vi "Single Tone Measurements.vi"(0 "scaled signals [EU]":waveform(dbl), 1 "tone detected":bool, 5 "frequency range":T1, 7 "window":T2 items=["None"=0, "Hanning"=1, "Hamming"=2, "Blackman-Harris"=3, "Exact Blackman"=4, "Blackman"=5, "Flat Top"=6, "4 Term B-Harris "=7, "7 Term B-Harris"=8, "Low Sidelobe"=9, "Force"=64, "Exponential"=65, "Blackman Nuttall"=11, "Triangle"=30, "Bartlett-Hanning"=31, "Bohman"=32, "Parzen"=33, "Welch"=34, "Kaiser"=60, "Dolph-Chebyshev"=61, "Gaussian"=62], 9 "Maximum Harmonic":i32, 11 "error in":errorcluster, 12 "Expected Frequency (Hz)":dbl) -> (4 "single-tone measurements":waveform(dbl)[](array[waveform]), 15 "error out":errorcluster)   [LabVIEW 2025, in "Tone Measurements.lvlib" / "Tone Measurements.lvclass"]
uses:
  Tone Measurements.lvclass
  <vilib>/addons/_NISVFA/_Shared subVIs/Controls/svc_Window.ctl
  <vilib>/addons/Sound and Vibration/svt_Level/SVL AC & DC Level (Time) (1 Ch).vi
  <vilib>/addons/Sound and Vibration/svt_Single Tone Measurements/SVT Spurious Free Dynamic Range (Frequency) (1 Ch).vi
  <vilib>/addons/_NISVFA/_Spectrum Processing/SVFA Unit Conversion (Complex) (1 Ch).vi
  <vilib>/addons/_NISVFA/_Spectrum Processing/SVFA Power in Band (1 Ch).vi
  <vilib>/addons/_NISVFA/_Shared subVIs/Common/svc_Get SV Channel Info.vi
  <vilib>/Analysis/baseanly.llb/Mean.vi
  <vilib>/Analysis/baseanly.llb/Mean (DBL).vi
  <vilib>/addons/_NISVFA/_Shared subVIs/Windowing/svfa_Scaled Time Domain Window (Array).vi
  <vilib>/addons/_NISVFA/_Spectrum Processing/SVFA Get Spectrum Subset.vi
  <vilib>/addons/_NISVFA/_Spectrum Processing/SVFA Get Spectrum Subset (Complex) (1 Ch).vi
  <vilib>/addons/_NISVFA/_Shared subVIs/Common/svc_Window Parameters.vi
  <vilib>/addons/_NISVFA/_Shared subVIs/Common/svc_Extract Single Tone Information (complex).vi
  <vilib>/addons/_NISVFA/_Shared subVIs/Common/svc_Check Frequency Range in Spectrum.vi
  <vilib>/addons/_NISVFA/_Spectrum Processing/SVFA Spectrum Peak Search.vi
  <vilib>/addons/_NISVFA/_Spectrum Processing/SVFA Spectrum Peak Search (1 Ch).vi
  <vilib>/addons/_NISVFA/_Shared subVIs/Common/svc_Spectrum Units.vi
  <vilib>/addons/_NISVFA/_Shared subVIs/Common/svc_Log View for Spectrum (1Ch).vi
  <vilib>/addons/_NISVFA/_Spectrum Processing/SVFA Unit Conversion (1 Ch).vi
  <vilib>/addons/_NISVFA/_Shared subVIs/Common/svc_Complex Datatype Defaults.vi
  <vilib>/addons/_NISVFA/_Spectrum Processing/SVFA Get Spectrum Subset (1 Ch).vi
  <vilib>/addons/_NISVFA/_Spectrum Processing/subVIs/svfa_Spectrum Info Window to windowTd Type Def.vi
  <vilib>/addons/_NISVFA/_Shared subVIs/Common/svc_Unit Label to Engineering Units.vi
  <vilib>/addons/_NISVFA/_Shared subVIs/Common/svc_Engineering Units to Unit Label.vi
  <vilib>/Analysis/4window.llb/Force Window.vi
  <vilib>/Analysis/4window.llb/Force Window (DBL).vi
  <vilib>/Analysis/4window.llb/Exponential Window.vi
  <vilib>/Analysis/4window.llb/Exponential Window (DBL).vi
  <vilib>/addons/_NISVFA/_Shared subVIs/Common/svc_Build Unit Label for Frequency Range.vi
  <vilib>/addons/_NISVFA/_Spectrum Processing/SVFA Get Tone Amplitude and Phase (1 Ch).vi
  <vilib>/addons/_NISVFA/_Spectrum Processing/subVIs/svfa_Compute Complex Spectrum for Export.vi
  <vilib>/addons/_NISVFA/_Shared subVIs/Common/svc_Check Frequency Range in Bandwidth.vi
  <vilib>/addons/_NISVFA/_Shared subVIs/Common/svc_Convert Start and Stop to Start Index and Length.vi
  <vilib>/addons/_NISVFA/_Spectrum Processing/subVIs/svfa_Spectrum Peak Search.vi
  <vilib>/addons/_NISVFA/_Shared subVIs/Common/svc_Format Value (DBL).vi
  <vilib>/addons/_NISVFA/_Shared subVIs/Common/svc_Get Weighting Enum and Labels.vi
  <vilib>/addons/_NISVFA/_Shared subVIs/Common/svc_Surround NonAlpha String with Parentheses.vi
  <vilib>/dlg_ctls.llb/Space Constant.vi
  <vilib>/addons/_NISVFA/_Shared subVIs/Common/svc_Unwrap Phase.vi
  <vilib>/addons/_NISVFA/_Shared subVIs/Common/svc_Convert Spectrum Array to dB.vi
  <vilib>/addons/_NISVFA/_Spectrum Processing/subVIs/svfa_Conversion Utility (spectrum info).vi
  <vilib>/addons/_NISVFA/_Spectrum Processing/subVIs/svfa_Window Frequency Response.vi
  <vilib>/addons/_NISVFA/_Spectrum Processing/subVIs/svfa_Window Frequency Response (double array).vi
  <vilib>/Analysis/baseanly.llb/Dot Product.vi
  <vilib>/Analysis/baseanly.llb/Complex Dot Product.vi
  <vilib>/addons/_NISVFA/_Spectrum Processing/subVIs/svfa_Peak Rough Search Indices.vi
  <vilib>/addons/_NISVFA/_Shared subVIs/Common/svc_Unit Label Lexical Class.vi
  <vilib>/addons/_NISVFA/_Spectrum Processing/subVIs/svfa_Peak to RMS to Peak2Peak.vi
  <vilib>/addons/_NISVFA/_Spectrum Processing/subVIs/svfa_Mag to Mag2.vi
  <vilib>/addons/_NISVFA/_Spectrum Processing/subVIs/svfa_Linear to dB.vi
  <vilib>/addons/_NISVFA/_Spectrum Processing/subVIs/svfa_dBrefA to dBrefB.vi
  <vilib>/addons/_NISVFA/_Spectrum Processing/subVIs/svfa_Spectrum to Spectral Density.vi
  <vilib>/addons/_NISVFA/_Spectrum Processing/subVIs/svfa_Rect Window Frequency Response.vi
  <vilib>/addons/_NISVFA/_Spectrum Processing/subVIs/svfa_Cosine Window Coefficients.vi
  <vilib>/addons/_NISVFA/_Shared subVIs/Common/svc_Get Window Info.vi
  <vilib>/Analysis/0measdsp.llb/Scaled Time Domain Window.vi
  <vilib>/Analysis/0measdsp.llb/Scaled Time Domain Window (DBL).vi
  <vilib>/Utility/error.llb/Error Cluster From Error Code.vi
  <vilib>/Analysis/baseanly.llb/Std Deviation and Variance.vi
  <vilib>/addons/_NISVFA/_Shared subVIs/Common/svc_Caller VI Returned in Error Source.vi
  <vilib>/addons/_NISVFA/_Baseband FFT/SVFA FFT Spectrum (Complex) (1 Ch).vi
  <vilib>/addons/Sound and Vibration/svt_Distortion/SVT THD and Harmonic Components (Time) (1 Ch).vi
  <vilib>/addons/Sound and Vibration/svt_Distortion/SVT SNR without Harmonics (Frequency) (1 Ch).vi
  <vilib>/addons/Sound and Vibration/svt_Distortion/subVIs/sv_Check Data Valid (Audio) (1 Ch).vi
  <vilib>/addons/_NISVFA/_Shared subVIs/Common/svc_Convert Frequency to Frequency String.vi
  <vilib>/Analysis/4window.llb/window parameters.vi
  <vilib>/Analysis/4window.llb/Window Properties.vi
  <vilib>/Analysis/4window.llb/Window Properties by Name.vi
  <vilib>/addons/_NISVFA/_Spectrum Processing/subVIs/svfa_Spectrum Peak Tone Search and Estimation (complex).vi
  <vilib>/measure/masignal.llb/Tones and Noise Waveform.vi
  <vilib>/addons/_NISVFA/_Shared subVIs/Common/svc_FFT with Window.vi
  <vilib>/Analysis/1siggen.llb/Square Wave.vi
  <vilib>/addons/_NISVFA/_Spectrum Processing/subVIs/svfa_Three Finger Peak Search.vi
  <vilib>/addons/Sound and Vibration/svt_Distortion/subVIs/sv_Peak View Amplitude (1 Ch).vi
  <vilib>/addons/Sound and Vibration/svt_Single Tone Measurements/SoundVib_SingleTone.lvlib
  <vilib>/addons/Sound and Vibration/svt_Distortion/SoundVib_Distortion.lvlib
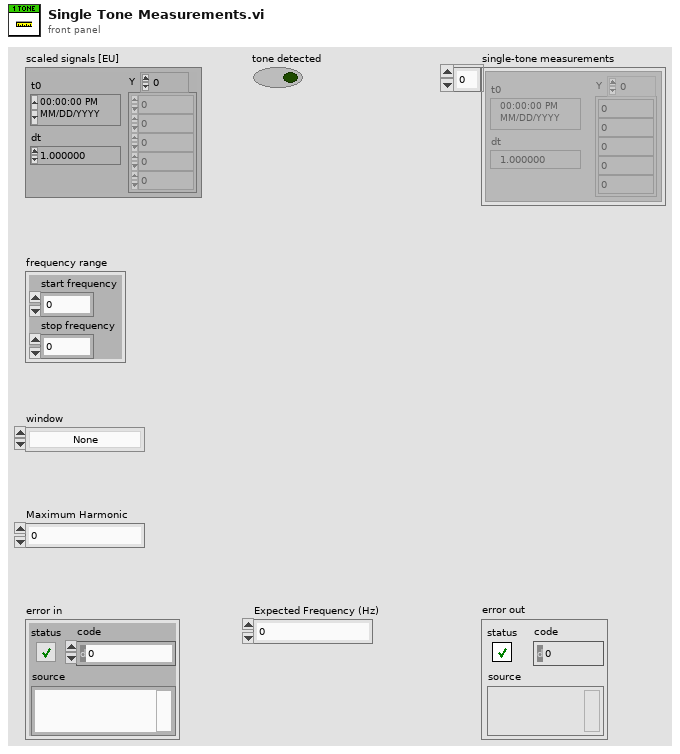
[diagram p1: front panel]
types:
  T1 = cluster{"start frequency":dbl, "stop frequency":dbl}
  T2 = typedef "svc_Window.ctl" = u32
  T3 = cluster{"linear/dB":enum16{"no change", "linear", "dB"}, "dB reference (0: no change)":dbl, "power/magnitude":enum16{"no change", "power", "magnitude"}, "view":enum16{"no change", "rms", "peak", "peak-peak"}}
  T4 = cluster{"spurious free dynamic range units":enum16{"dB", "ENOB"}, "detected fundamental amplitude units":enum16{"EU rms", "EU peak", "EU peak-peak"}, "dB reference for detected peaks":enum16{"fundamental", "dB ref"}}
  T5 = cluster{"SNR units":enum16{"dB", "linear ratio", "%"}, "detected fundamental amplitude units":enum16{"EU rms", "EU peak", "EU peak-peak"}}
  T6 = cluster{"THD units":enum16{"dB", "linear ratio", "%"}, "harmonic component amplitude units":enum16{"EU rms", "EU peak", "EU peak-peak", "dB ref fund"}, "detected fundamental amplitude units":enum16{"EU rms", "EU peak", "EU peak-peak"}}
  T7 = typedef "svc_Spectrum Info.ctl" = cluster{"channel name":string, "description":string, "x-axis units":T8, "spectral info":cluster{"spectrum type":T9, "linear/dB":enum16{"linear", "dB"}, "window":u16, "window size":i32, "FFT size":i32}, "engineering units":T10, "custom label":string, "dB reference [EU]":dbl, "peak units":enum16{"rms", "peak", "peak-peak"}, "weighting filter":T11, "spectral density?":bool, "unit label":string, "spectrum skewed?":bool, "complimentary spectrum units":T12}
  T8 = typedef "svc_X-Axis Units.ctl" = u16
  T9 = typedef "svc_Spectrum Type.ctl" = enum16{"FFT Spectrum [complex]", "Amplitude [Magnitude]", "Power [Magnitude^2]", "Cross Spectrum [complex]", "Frequency Response [Complex]"}
  T10 = typedef "svc_Engineering Units Text Ring.ctl" = u16
  T11 = typedef "svc_Weighting Filter Text Ring.ctl" = u16
  T12 = typedef "svc_Complimentary Spectrum Units.ctl" = enum16{"none", "radians", "degrees", "cycles", "imaginary"}
  T13 = cluster{"complex spectrum response":cluster{"f0":dbl, "df":dbl, "complex spectrum":cdb[]}, "spectrum info":T7}
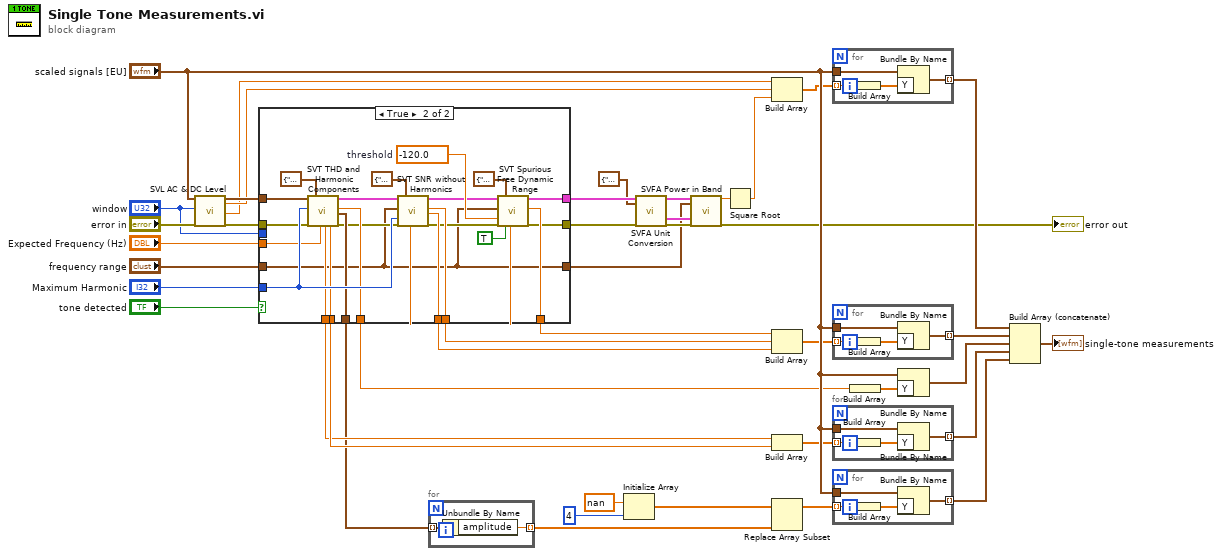
[diagram p0: block diagram]
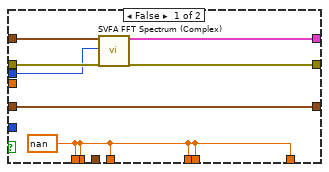
[diagram p2: hidden frame]
diagram:
  n1 = call-poly <vilib>:"SVL AC & DC Level.vi"("scaled signal [EU]"="scaled signals [EU]", "window"="window", "error in (no error)"="error in") -> ("AC signal [EU]"=w38:waveform(dbl), "AC level [EU rms]"=w27:dbl, "DC level [EU]"=w26:dbl, "error out"=w39:errorcluster)  [unwired: 11 in, 2 out]
  n2 = case shown="True" "tone detected" {
    tunnel: "Maximum Harmonic" -> [_ w73]
    tunnel: "Expected Frequency (Hz)" -> [_ w72]
    tunnel: w39 -> [w49 w71]
    tunnel: w38 -> [w50 w70]
    tunnel: [w45 w69] -> w37
    tunnel: [w45 w68] -> w36
    tunnel: [w45 w66] -> w32
    tunnel: [w45 w65] -> w31
    tunnel: [w45 w64] -> w30
    tunnel: [_ w63] -> w19
    tunnel: [w45 w62] -> w16
    tunnel: [w46 w53] -> w13
    tunnel: [w47 w52] -> w12
    tunnel: "frequency range" -> [w44 w51]
    tunnel: "window" -> [w48 _]
    tunnel: [w44 w51] -> w1
    frame False {
      w45 = nan ("detected fundamental\nfrequency [Hz]")
      n3 = call-poly <vilib>:"SVFA FFT Spectrum (Complex).vi"("scaled signal [EU]"=w50, "window"=w48, "error in"=w49) -> ("complex spectrum"=w47:T13, "error out"=w46:errorcluster)  [unwired: 13 in, 2 out]
    }
    frame True {
      w67 = -120.0  # threshold
      n4 = call-poly <vilib>:"SVT THD and Harmonic Components.vi"("scaled signal [EU]"=w70, "maximum harmonic"=w73, "error in (no error)"=w71, "desired units"=T6 {"THD units"=enum."dB", "harmonic component amplitude units"=enum."EU peak", "detected fundamental amplitude units"=enum."EU peak"}, "expected fundamental frequency [Hz]"=w72) -> ("detected fundamental\nfrequency [Hz]"=w68:dbl, "detected fundamental\namplitude"=w69:dbl, "complex spectrum"=w57:T13, "THD"=w62:dbl, "harmonic components"=w63:cluster{"frequency [Hz]":dbl, "amplitude":dbl}[], "error out"=w55:errorcluster)  [unwired: 7 in, 2 out]
      n5 = call-poly <vilib>:"SVT SNR without Harmonics.vi"("complex spectrum"=w57, "frequency range"=w51, "maximum harmonic"=w73, "error in (no error)"=w55, "desired units"=T5 {"SNR units"=enum."dB", "detected fundamental amplitude units"=enum."EU rms"}, "expected fundamental frequency [Hz]"=w68) -> ("complex spectrum"=w56:T13, "SNR (without harmonics)"=w65:dbl, "SINAD"=w66:dbl, "error out"=w54:errorcluster)  [unwired: 6 in, 4 out]
      n6 = call-poly <vilib>:"SVT Spurious Free Dynamic Range.vi"("complex spectrum"=w56, "frequency range"=w51, "threshold [dBc]"=w67, "error in (no error)"=w54, "desired units"=T4 {"spurious free dynamic range units"=enum."dB", "detected fundamental amplitude units"=enum."EU peak", "dB reference for detected peaks"=enum."dB ref"}, "exclude harmonics"=TRUE, "expected fundamental\nfrequency [Hz]"=w68) -> ("complex spectrum"=w52:T13, "spurious free dynamic range"=w64:dbl, "error out"=w53:errorcluster)  [unwired: 5 in, 5 out]
    }
  }
  n7 = for {
    tunnel: w19 -> [w75] mode=indexing
    tunnel: [w74] -> w22 mode=indexing
    n8 = Unbundle By Name(w75) -> ("amplitude"=w74:dbl)
  }
  n9 = Initialize Array(nan ("element"), 4 ("dimension size")) -> (w23:dbl[])
  n10 = call-poly <vilib>:"SVFA Unit Conversion.vi"("complex spectrum"=w12, "desired scaling"=T3 {"linear/dB"=enum."no change", "dB reference (0: no change)"=0.0, "power/magnitude"=enum."power", "view"=enum."no change"}, "error in (no error)"=w13) -> ("converted spectrum"=w9:cluster{"x0":dbl, "dx":dbl, "magnitude":dbl[]}, "spectrum info out"=w8:T7, "error out"=w11:errorcluster)  [unwired: 11 in, 3 out]
  n11 = call-poly <vilib>:"SVFA Power in Band.vi"("spectrum"=w9, "range"=w1, "spectrum info"=w8, "error in (no error)"=w11) -> ("power in band"=w6:dbl, "error out"=→"error out":errorcluster)  [unwired: 13 in, 1 out]
  n12 = Square Root(x=w6) -> (sqrt(x)=w5:dbl)
  n13 = Build Array(w26, w27, w5) -> (w28:dbl[])
  n14 = Build Array(w30, w31, w32) -> (w33:dbl[])
  n15 = Build Array(w36, w37) -> (w25:dbl[])
  n16 = Replace Array Subset(array=w23, new element=w22) -> (w24:dbl[])  [unwired: 1 in]
  n17 = for {
    tunnel: [w78] -> w29 mode=indexing
    tunnel: w28 -> [w77] mode=indexing
    tunnel: "scaled signals [EU]" -> [w76]
    n18 = Build Array(w77) -> (w79:dbl[])
    n19 = Bundle By Name(cluster=w76, "Y"=w79) -> (w78:waveform(dbl))
  }
  n20 = for {
    tunnel: [w82] -> w34 mode=indexing
    tunnel: w33 -> [w81] mode=indexing
    tunnel: "scaled signals [EU]" -> [w80]
    n21 = Build Array(w81) -> (w83:dbl[])
    n22 = Bundle By Name(cluster=w80, "Y"=w83) -> (w82:waveform(dbl))
  }
  n23 = for {
    tunnel: [w86] -> w35 mode=indexing
    tunnel: w25 -> [w85] mode=indexing
    tunnel: "scaled signals [EU]" -> [w84]
    n24 = Build Array(w85) -> (w87:dbl[])
    n25 = Bundle By Name(cluster=w84, "Y"=w87) -> (w86:waveform(dbl))
  }
  n26 = for {
    tunnel: "scaled signals [EU]" -> [w90]
    tunnel: [w89] -> w18 mode=indexing
    tunnel: w24 -> [w88] mode=indexing
    n27 = Build Array(w88) -> (w91:dbl[])
    n28 = Bundle By Name(cluster=w90, "Y"=w91) -> (w89:waveform(dbl))
  }
  n29 = Build Array(w16) -> (w15:dbl[])
  n30 = Bundle By Name ("Build Waveform")(cluster="scaled signals [EU]", "Y"=w15) -> (w17:waveform(dbl))
  n31 = Build Array (concatenate)(w29, w34, w17, w35, w18) -> (→"single-tone measurements":waveform(dbl)[])
